vi "Get CMM Value.vi"(10 "CMM Table":dbl[][](array[numeric]), 11 "TT1-Deg F C.11":dbl) -> (3 "Value Out":dbl)   [LabVIEW 2018, in "RT - Analysis.lvlib"]
uses:
  RT - Analysis.lvlib
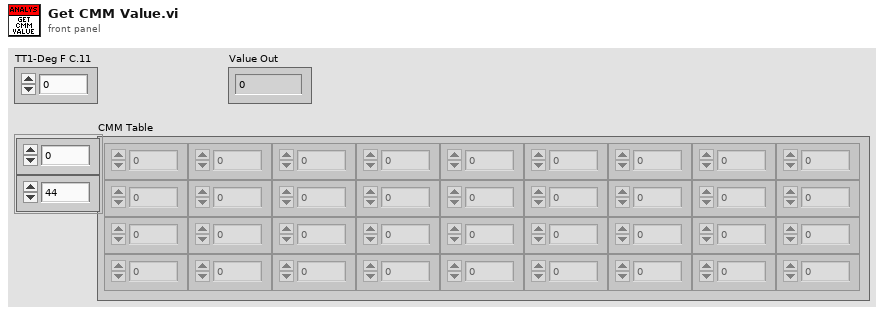
[diagram p1: front panel]
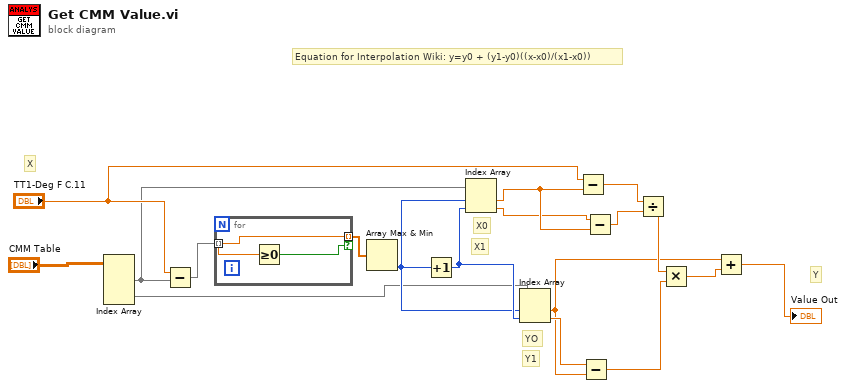
[diagram p0: block diagram]
diagram:
  # "Y"
  # "X"
  # "Y1"
  # "YO"
  # "X1"
  # "X0"
  # "Equation for Interpolation Wiki: y=y0 + (y1-y0)((x-x0)/(x1-x0))"
  n1 = Index Array(array="CMM Table") -> (element #1=w2:dbl[], element #2=w1:dbl[])  [unwired: 4 in]
  n2 = Subtract(x="TT1-Deg F C.11", y=w2) -> (x-y=w6:dbl[])
  n3 = for {
    tunnel: w6 -> [w20] mode=indexing
    tunnel: [w20] -> w5 mode=indexing if=w19
    n4 = Greater Or Equal To 0?(x=w20) -> (x >= 0?=w19:bool)
  }
  n5 = Array Max & Min(array=w5) -> (min index (indices)=w3:i32)  [unwired: 3 out]
  n6 = Increment(x=w3) -> (x+1=w4:i32)
  n7 = Index Array(array=w2, index #1=w3, index #2=w4) -> (element #1=w15:dbl, element #2=w7:dbl)
  n8 = Index Array(array=w1, index #1=w3, index #2=w4) -> (element #1=w10:dbl, element #2=w17:dbl)
  n9 = Subtract(x="TT1-Deg F C.11", y=w15) -> (x-y=w14:dbl)
  n10 = Subtract(x=w17, y=w10) -> (x-y=w11:dbl)
  n11 = Subtract(x=w7, y=w15) -> (x-y=w13:dbl)
  n12 = Divide(x=w14, y=w13) -> (x/y=w12:dbl)
  n13 = Multiply(x=w12, y=w11) -> (x*y=w9:dbl)
  n14 = Add(x=w10, y=w9) -> (x+y=→"Value Out":dbl)
